vi "examen123.vi"() -> ()   [LabVIEW 2020]
panel:
  out "#PROCESOS":i32
  in  "MENU F.T.":enum16{"SENO", "COSENO", "TANGENTE"}(ring)
  in  "MENÙ P.":T1(ring)
  in  "PARAR":bool
  out "RESULTADO":dbl
  in  "CIFRA 2":dbl
  in  "CIFRA 1":dbl format="%#_3g"
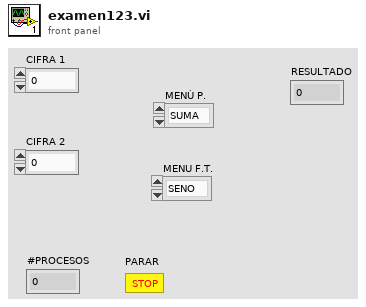
[diagram p1: front panel]
types:
  T1 = enum16{"SUMA", "RESTA", "MULTIPLICACION", "DIVISION", "EXPONENTE", "RAIZ", "FUNCIONES TRIGONOMETRICAS", "GRADOS A RADIANES", "RADIANES A GRADOS"}
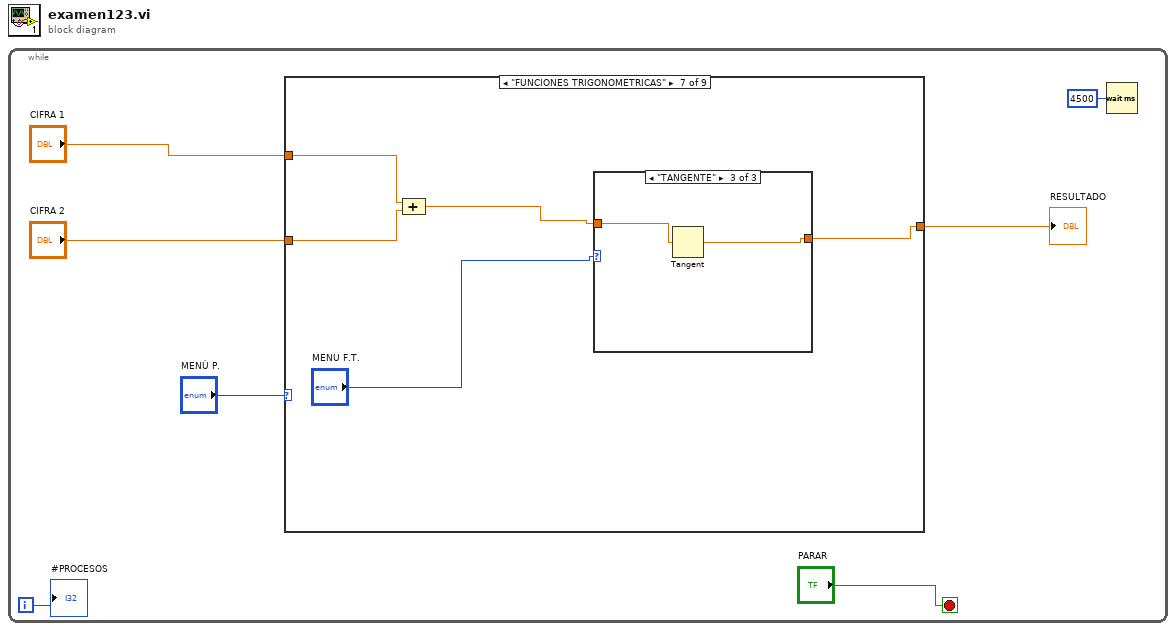
[diagram p0: block diagram]
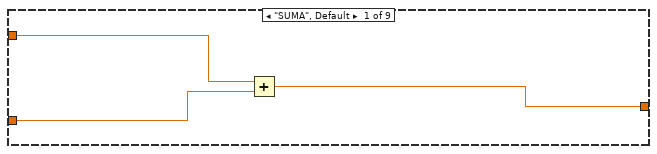
[diagram p2: hidden frame]
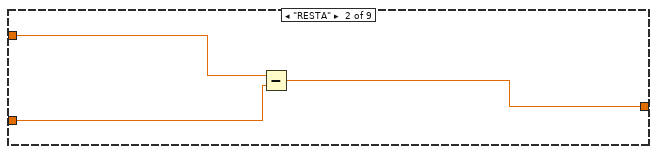
[diagram p3: hidden frame]
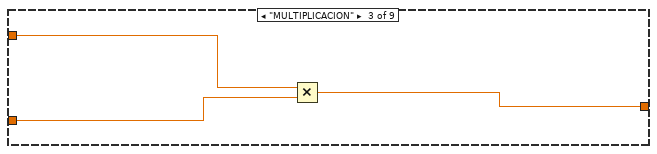
[diagram p4: hidden frame]
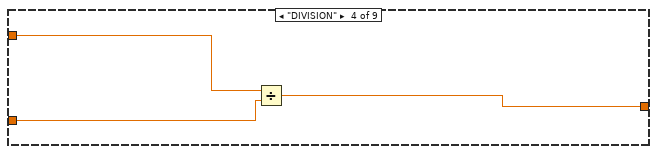
[diagram p5: hidden frame]
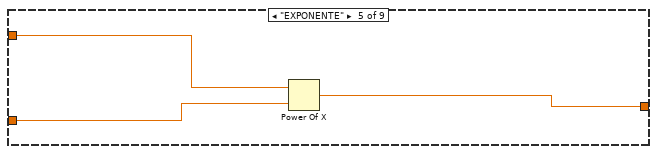
[diagram p6: hidden frame]
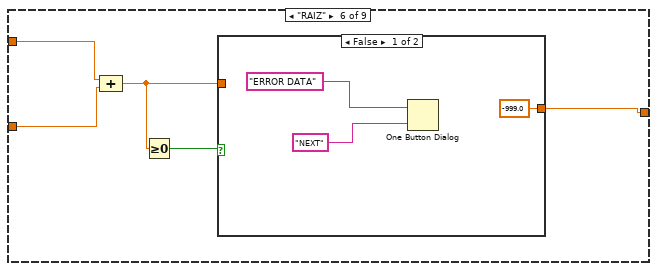
[diagram p7: hidden frame]
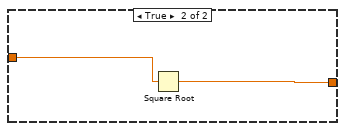
[diagram p8: hidden frame]
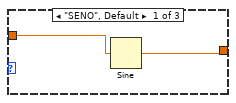
[diagram p9: hidden frame]
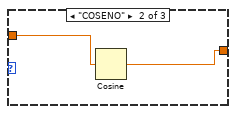
[diagram p10: hidden frame]
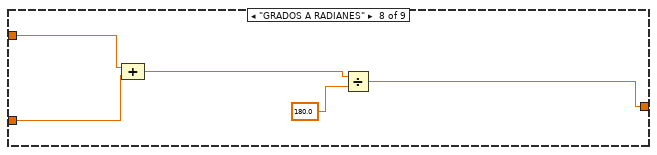
[diagram p11: hidden frame]
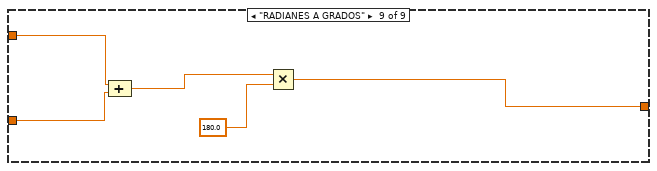
[diagram p12: hidden frame]
diagram:
  n1 = while {
    i -> [w2]
    stop <- "PARAR" stop-if-true
    n2 = case shown="\"FUNCIONES TRIGONOMETRICAS\"" "MENÙ P." {
      tunnel: "CIFRA 1" -> [w10 w13 w16 w19 w22 w26 w37 w47 w53]
      tunnel: [w9 w12 w15 w18 w21 w27 w33 w44 w50] -> w4
      tunnel: "CIFRA 2" -> [w8 w11 w14 w17 w20 w25 w36 w46 w52]
      frame "SUMA", Default {
        n3 = Add(x=w10, y=w8) -> (x+y=w9:dbl)
      }
      frame "RESTA" {
        n4 = Subtract(x=w13, y=w11) -> (x-y=w12:dbl)
      }
      frame "MULTIPLICACION" {
        n5 = Multiply(x=w16, y=w14) -> (x*y=w15:dbl)
      }
      frame "DIVISION" {
        n6 = Divide(x=w19, y=w17) -> (x/y=w18:dbl)
      }
      frame "EXPONENTE" {
        n7 = Power Of X(1:w20, 2:w22) -> (0:w21:dbl)
      }
      frame "RAIZ" {
        n8 = Compound Arithmetic op=ADD(w26, w25) -> (w23:dbl)
        n9 = Greater Or Equal To 0?(x=w23) -> (x >= 0?=w24:bool)
        n10 = case shown="False" w24 {
          tunnel: [-999.0 w32] -> w27
          tunnel: w23 -> [_ w31]
          frame False {
            n11 = One Button Dialog(message="ERROR DATA", button name ("OK")="NEXT") -> ()  [unwired: 1 out]
          }
          frame True {
            n12 = Square Root(x=w31) -> (sqrt(x)=w32:dbl)
          }
        }
      }
      frame "FUNCIONES TRIGONOMETRICAS" {
        n13 = Compound Arithmetic op=ADD(w37, w36) -> (w34:dbl)
        n14 = case shown="\"TANGENTE\"" "MENU F.T." {
          tunnel: w34 -> [w39 w41 w43]
          tunnel: [w38 w40 w42] -> w33
          frame "SENO", Default {
            n15 = Sine(x=w39) -> (sin(x)=w38:dbl)
          }
          frame "COSENO" {
            n16 = Cosine(x=w41) -> (cos(x)=w40:dbl)
          }
          frame "TANGENTE" {
            n17 = Tangent(1:w43) -> (0:w42:dbl)
          }
        }
      }
      frame "GRADOS A RADIANES" {
        n18 = Compound Arithmetic op=ADD(w47, w46) -> (w45:dbl)
        n19 = Divide(x=w45, y=180.0) -> (x/y=w44:dbl)
      }
      frame "RADIANES A GRADOS" {
        n20 = Compound Arithmetic op=ADD(w53, w52) -> (w51:dbl)
        n21 = Multiply(x=w51, y=180.0) -> (x*y=w50:dbl)
      }
    }
    "RESULTADO" <- w4
    n22 = Wait (ms)(milliseconds to wait=u32 4500) -> ()  [unwired: 1 out]
    "#PROCESOS" <- w2
  }
